vi "Global_datareceivefromC#.vi"(8 "ArrayIN":T1[](array[typedef]), 11 "OP":enum16{"ini", "read", "write"}(ring)) -> (0 "Array":T1[](array[typedef]))   [LabVIEW 2015]
uses:
  c#aoiresultctl.ctl
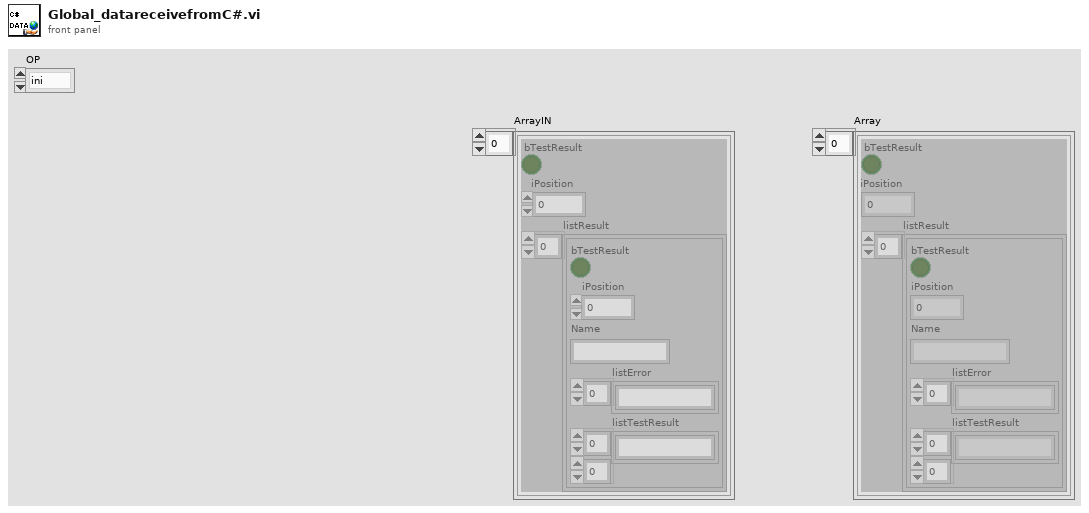
[diagram p1: front panel]
types:
  T1 = typedef "c#aoiresultctl.ctl" = cluster{"bTestResult":bool, "iPosition":dbl, "listResult":cluster{"bTestResult":bool, "iPosition":dbl, "Name":string, "listError":string[], "listTestResult":string[][]}[]}
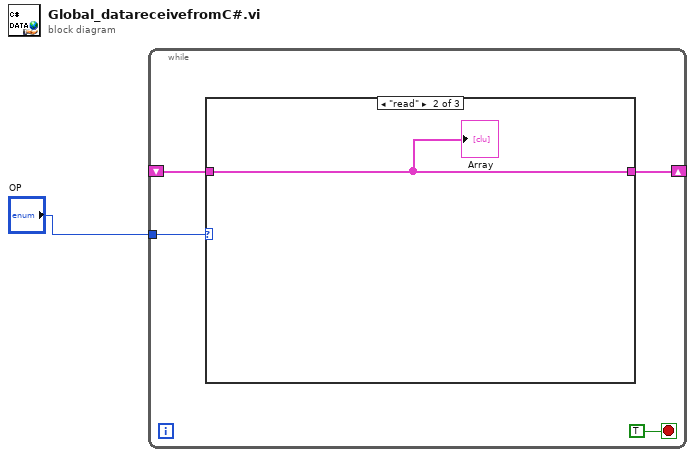
[diagram p0: block diagram]
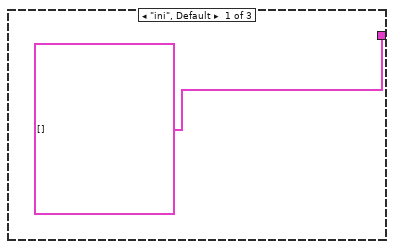
[diagram p2: hidden frame]
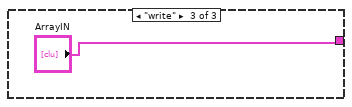
[diagram p3: hidden frame]
diagram:
  n1 = while {
    tunnel: "OP" -> [w5]
    shift-right: [w4] -> _
    shift-left: _ -> [w3]
    stop <- TRUE stop-if-true
    n2 = case shown="\"read\"" w5 {
      tunnel: [T1[] [] w7 "ArrayIN"] -> w4
      tunnel: w3 -> [_ w7 _]
      frame "ini", Default {
      }
      frame "read" {
        "Array" <- w7
      }
      frame "write" {
      }
    }
  }
